vi "Compose Array - 2D Array - Returns Array.vi"() -> ()   [LabVIEW 2017, in "Composition.Tests.lvlib"]
uses:
  Composition.Tests.lvlib
  9c0ba3b4-1cb7-4f02-a971-025ef2be0526.vi
  <vilib>/addons/_JKI Toolkits/Caraya/classes/Assert/Assert Equal Value_Variant.vi
  <vilib>/addons/_JKI Toolkits/Caraya/classes/Test/Test.lvclass
  <vilib>/addons/_JKI Toolkits/Caraya/classes/Assert/Assert.lvclass
panel:
  out "error out":errorcluster
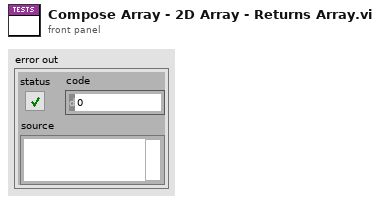
[diagram p1: front panel]
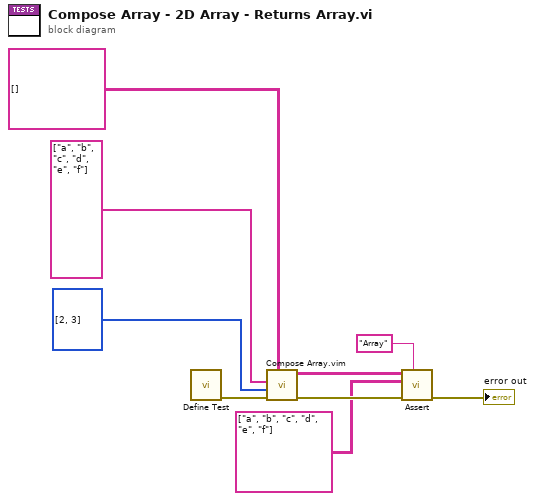
[diagram p0: block diagram]
diagram:
  n1 = call <vilib>:"Define Test.vi"() -> ("error out"=w7:errorcluster)  [unwired: 10 in, 1 out]
  n2 = call "Compose Array.vim"("Array Type"=string[][] [], "error in (no error)"=w7, "Dimension Sizes"=i32[] [2, 3], "Elements"=string[] ["a", "b", "c", "d", "e", "f"]) -> ("error out"=w5:errorcluster, "Array"=w3:string[][])  [unwired: 6 in]
  n3 = call-poly <vilib>:"Assert.vi"("Label"="Array", "error in (no error)"=w5, "Y"=string[][] [["a", "b", "c"], ["d", "e", "f"]], "X"=w3) -> ("error out"=→"error out":errorcluster)  [unwired: 6 in, 1 out]
